vi "Add to Mean.vi"(10 "Non Object":refnum<class "JSON Value.lvclass">, 11 "JSON Value In":refnum<class "JSON Value.lvclass">) -> (3 "JSON Mean out":refnum<class "JSON Running Mean.lvclass">)   [LabVIEW 2020, in "Library Commun.lvlib" / "JSON Value.lvclass"]
uses:
  JSON Value.lvclass
  JSON Running Mean/JSON Running Mean.lvclass
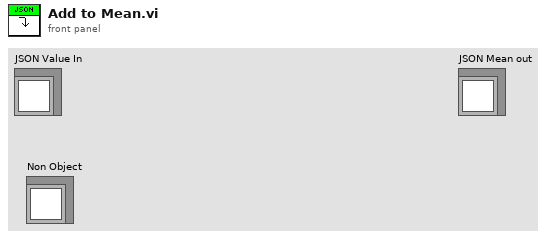
[diagram p1: front panel]
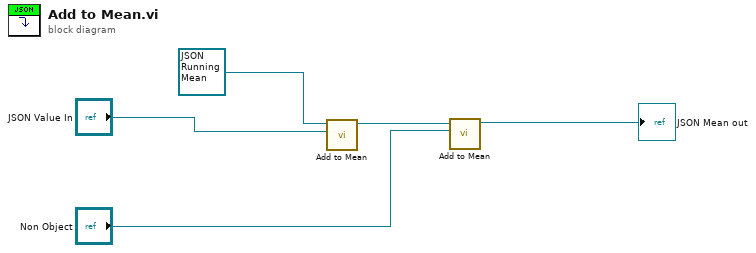
[diagram p0: block diagram]
diagram:
  n1 = call-dynamic "Add to Mean.vi"("Non Object"="JSON Value In", "JSON Running Mean In"=refnum<class "JSON Running Mean.lvclass"> refnum ("JSON Running Mean.lvclass")) -> ("JSON Running Mean"=w3:refnum<class "JSON Running Mean.lvclass">)  [unwired: 9 in]
  n2 = call-dynamic "Add to Mean.vi"("Non Object"="Non Object", "JSON Running Mean In"=w3) -> ("JSON Running Mean"=→"JSON Mean out":refnum<class "JSON Running Mean.lvclass">)  [unwired: 9 in]
